vi "MAINKLEURECHTWEL.vi"() -> ()   [LabVIEW 2018]
doc: "Use this template to build a standard state machine design pattern. Each state executes code and determines which state to transition to. Contrast this design pattern with the User Interface Event Handler pattern, in which code executes in response to user actions. Contrast this design pattern also with the Queued Message Handler pattern, in which each message handling code can queue zero or more new messages."
uses:
  FSM States.ctl
panel:
  in  "Kleurmaken":bool
  out "Beginning State":T1
  in  "stop":bool
  in  "digital out":bool[](array[boolean])
  in  "KLEUREN":bool
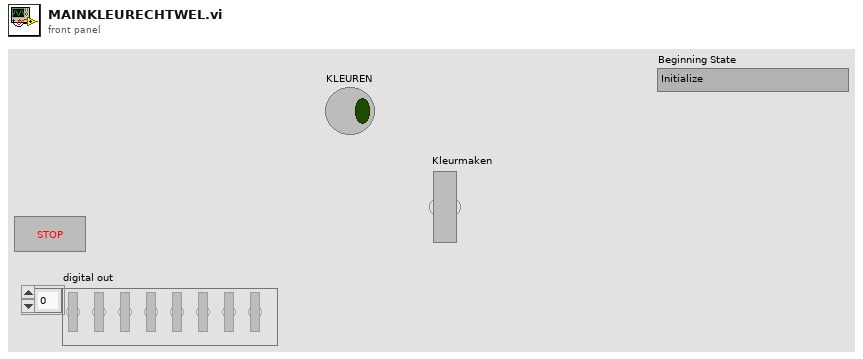
[diagram p1: front panel]
types:
  T1 = typedef "FSM States.ctl" = enum16{"Initialize", "ROOD", "GROEN ", "Blauw "}
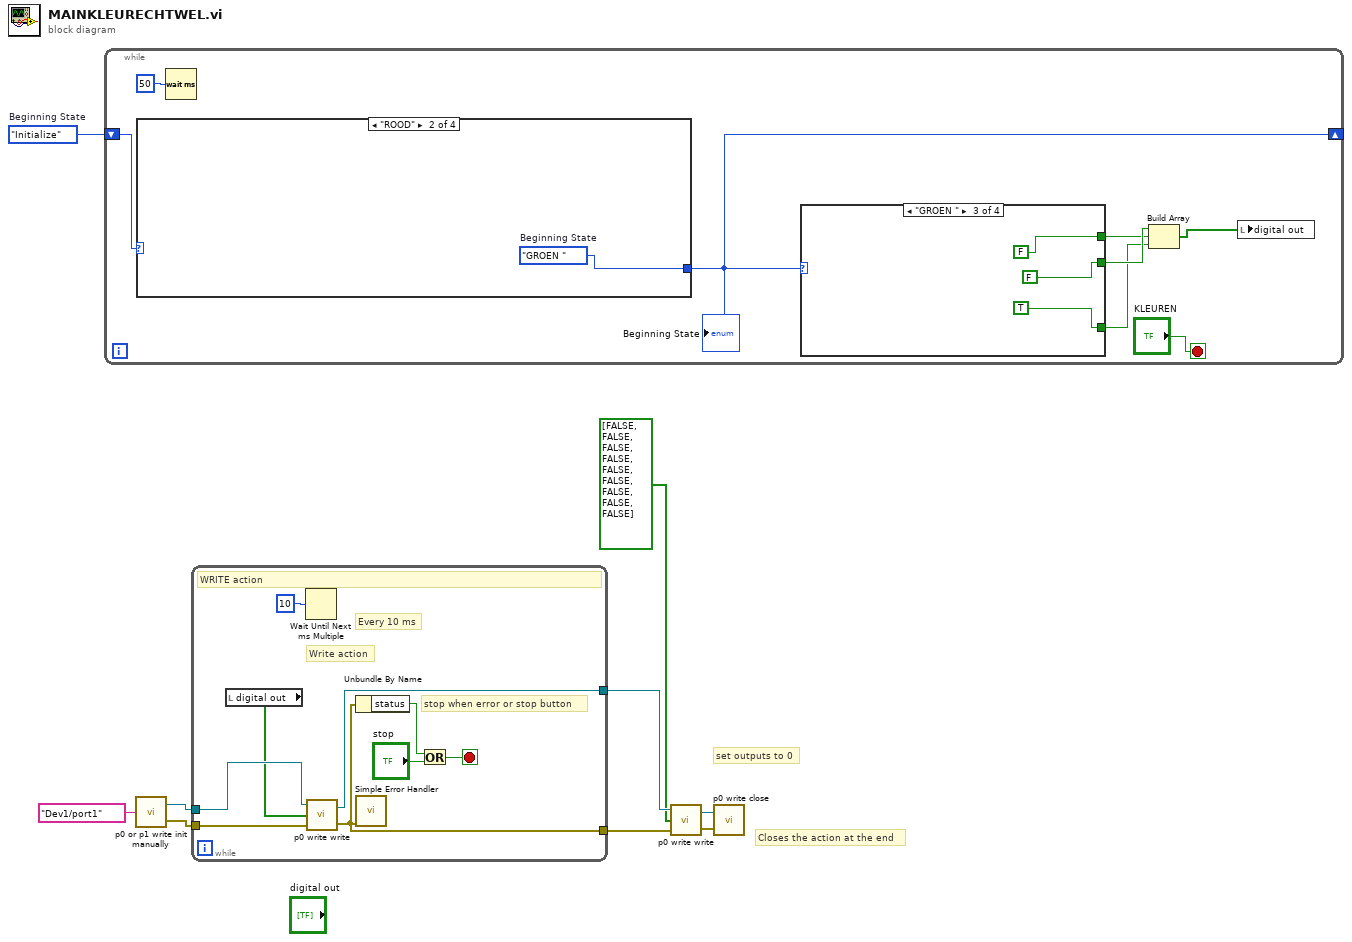
[diagram p0: block diagram]
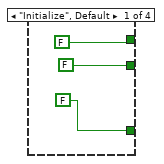
[diagram p2: hidden frame]
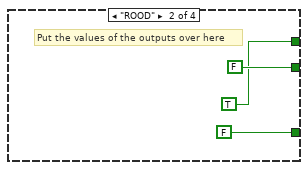
[diagram p3: hidden frame]
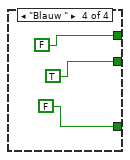
[diagram p4: hidden frame]
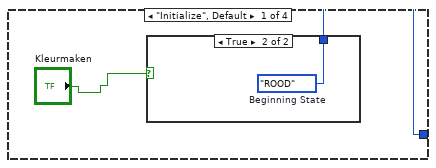
[diagram p5: hidden frame]
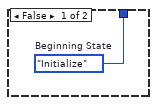
[diagram p6: hidden frame]
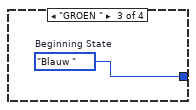
[diagram p7: hidden frame]
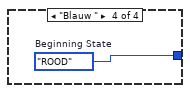
[diagram p8: hidden frame]
diagram:
  w9 = FSM_States."Initialize"  # Beginning State
  # "set outputs to 0"
  # "Closes the action at the end"
  n1 = while {
    shift-right: [w10] -> _
    shift-left: w9 -> [w17]
    stop <- "KLEUREN" stop-if-true
    n2 = case shown="\"ROOD\"" w17 {
      tunnel: [w31 w34 w35 w36] -> w10
      frame "Initialize", Default {
        n3 = case shown="True" "Kleurmaken" {
          tunnel: [w32 w33] -> w31
          frame False {
            w32 = FSM_States."Initialize"  # Beginning State
          }
          frame True {
            w33 = FSM_States."ROOD"  # Beginning State
          }
        }
      }
      frame "ROOD" {
        w34 = FSM_States."GROEN "  # Beginning State
      }
      frame "GROEN " {
        w35 = FSM_States."Blauw "  # Beginning State
      }
      frame "Blauw " {
        w36 = FSM_States."ROOD"  # Beginning State
      }
    }
    "Beginning State" <- w10
    n4 = Wait (ms)(milliseconds to wait=u32 50) -> ()  [unwired: 1 out]
    n5 = case shown="\"GROEN \"" w10 {
      tunnel: [FALSE FALSE FALSE TRUE] -> w13
      tunnel: [FALSE TRUE FALSE FALSE] -> w12
      tunnel: [FALSE FALSE TRUE FALSE] -> w11
      frame "Initialize", Default {
      }
      frame "ROOD" {
        # "Put the values of the outputs over here"
      }
      frame "GROEN " {
      }
      frame "Blauw " {
      }
    }
    n6 = Build Array(w13, w12, w11) -> (w14:bool[])
    n7 = local write "digital out"(w14) -> ()
  }
  n8 = call "p0 or p1 write init manually.vi"("Port"=tag "Dev1/port1") -> ("task out"=w3:refnum<k21>, "error out"=w2:errorcluster)
  n9 = while {
    tunnel: w3 -> [w45]
    tunnel: [w44] -> w8
    tunnel: w2 -> [w43]
    tunnel: [w39] -> w7
    stop <- w40 stop-if-true
    # "stop when error or stop button"
    # "Every 10 ms"
    # "Write action"
    # "WRITE action"
    n10 = local read "digital out"() -> (w37:bool[])
    n11 = Wait Until Next ms Multiple(millisecond multiple=u32 10) -> ()  [unwired: 1 out]
    n12 = call "p0 write write.vi"("error in"=w43, "digital out"=w37, "task/channels in"=w45) -> ("error out"=w39:errorcluster, "task out"=w44:refnum<k21>)
    n13 = Unbundle By Name(w39) -> ("status"=w38:bool)
    n14 = call <vilib>:"Simple Error Handler.vi"("error in (no error)"=w39) -> ()  [unwired: 4 in, 5 out]
    n15 = Or(x=w38, y="stop") -> (x .or. y?=w40:bool)
  }
  n16 = call "p0 write write.vi"("error in"=w7, "digital out"=bool[] [FALSE, FALSE, FALSE, FALSE, FALSE, FALSE, FALSE, FALSE, FALSE], "task/channels in"=w8) -> ("error out"=w5:errorcluster, "task out"=w6:refnum<k21>)
  n17 = call "p0 write close.vi"("error in"=w5, "task/channels in"=w6) -> ()
